vi "PXI-2510 Fault Bus Page.vi"(8 "error in (no error)":errorcluster, 11 "Node Ptr":T2 format="%.0x") -> (0 "error out":errorcluster)   [LabVIEW 2020, in "PXI-2510 System Explorer.lvlib"]
uses:
  PXI-2510 System Explorer.lvlib
  <vilib>/NI VeriStand/Custom Device API/Custom Device Item Ref.ctl
  Shared/Fault Bus Input Selector.ctl
  <vilib>/NI VeriStand/Custom Device API/Custom Device API.lvlib
panel:
  in  "Fault Bus Input Selector Default Value":T1=enum."Input 0"
  in  "Header":cluster{"Section Name":string}={"Section Name"="Custom Device Item Settings"}
  in  "Description":string
  in  "Name":string
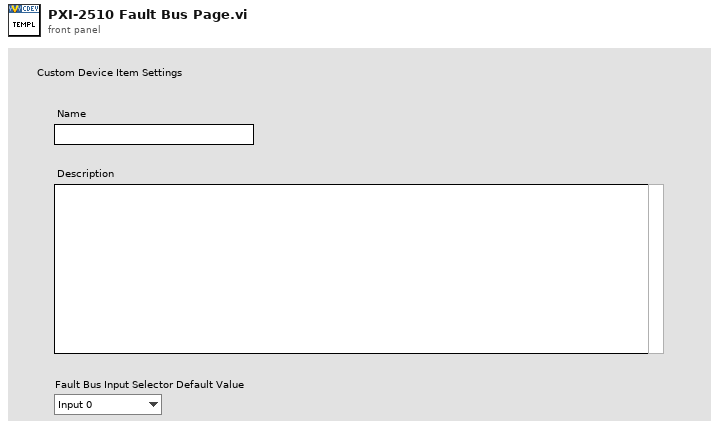
[diagram p1: front panel]
types:
  T1 = typedef "Fault Bus Input Selector.ctl" = enum16{"Default", "Input 0", "Input 1", "Input 2", "Input 3", "Main Bus Only"}
  T2 = typedef "Custom Device API.lvlib/Custom Device Item Ref.ctl" = u64
  T3 = typedef "Custom Device API.lvlib/Custom Device Item Info.ctl" = cluster{"Name":string, "Is Channel":bool, "GUID":string, "Is Waveform":bool}
  T4 = typedef "Custom Device API.lvlib/Custom Device Channel.ctl" = cluster{"Type":T5, "Units":string, "Default Value":dbl, "Faultable":bool, "Scalable":bool}
  T5 = typedef "Custom Device API.lvlib/Custom Device Channel Type.ctl" = enum16{"Input", "Output"}
  T6 = typedef "Custom Device API.lvlib/Custom Device Commands.ctl" = enum16{"Default", "Item renamed", "Shutdown", "Dynamic button pressed"}
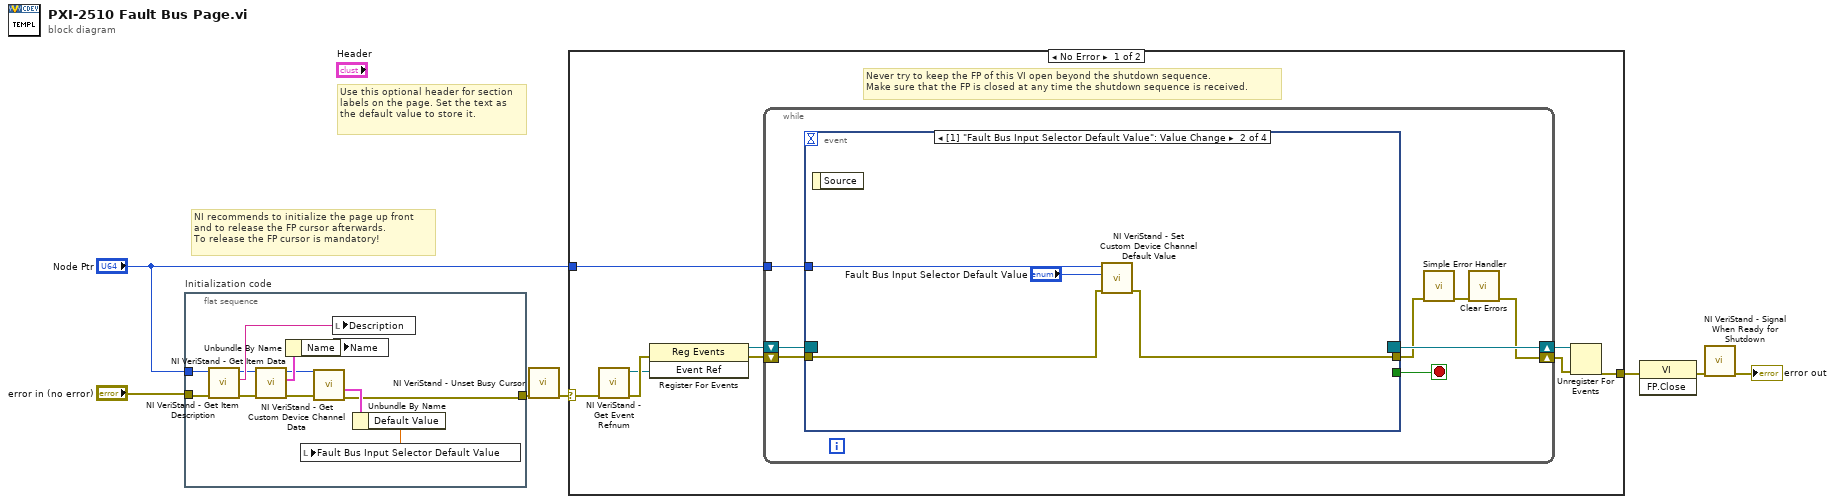
[diagram p0: block diagram]
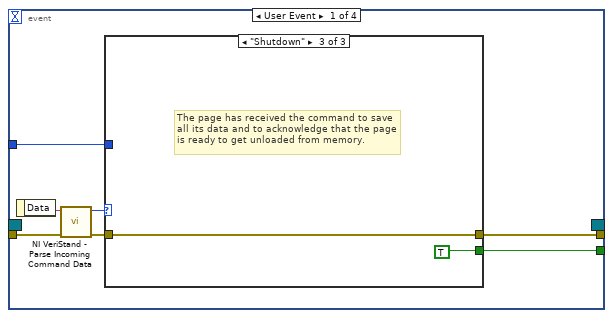
[diagram p2: hidden frame]
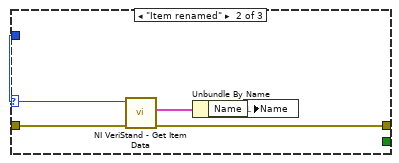
[diagram p4: hidden frame]
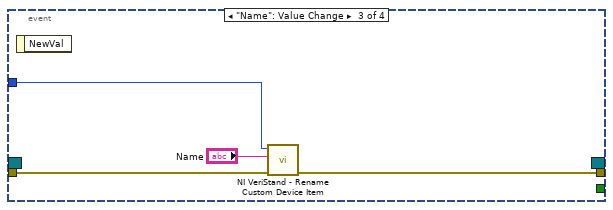
[diagram p5: hidden frame]
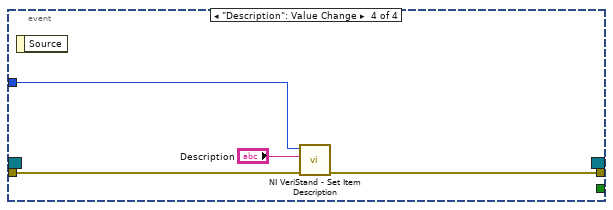
[diagram p6: hidden frame]
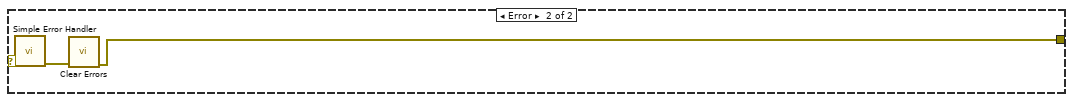
[diagram p7: hidden frame]
diagram:
  # "Use this optional header for section labels on the page. Set the text as the default value to store it."
  # "NI recommends to initialize the page up front\nand to release the FP cursor afterwards.\nTo release the FP cursor is mandatory!"
  n1 = flat-sequence "Initialization code" {
    tunnel: "error in (no error)" -> [w19]
    tunnel: "Node Ptr" -> [w18]
    tunnel: [w8] -> w2
    frame #0 {
      n2 = call <vilib>:"NI VeriStand - Get Item Description.vi"("error in (no error)"=w19, "Item Ref in"=w18) -> ("error out"=w16:errorcluster, "Description"=w17:string, "Item Ref out"=w15:T2)  [unwired: 7 out]
      n3 = call <vilib>:"NI VeriStand - Get Item Data.vi"("error in (no error)"=w16, "Item Ref in"=w15) -> ("error out"=w11:errorcluster, "Item Info"=w14:T3, "Item Ref out"=w12:T2)  [unwired: 7 out]
      n4 = Unbundle By Name(w14) -> ("Name"=w13:string)
      n5 = call <vilib>:"NI VeriStand - Get Custom Device Channel Data.vi"("error in (no error)"=w11, "Channel Ref in"=w12) -> ("error out"=w8:errorcluster, "Channel"=w10:T4)  [unwired: 4 in, 4 out]
      n6 = local write "Description"(w17) -> ()
      n7 = local write "Name"(w13) -> ()
      n8 = Unbundle By Name(w10) -> ("Default Value"=w9:dbl)
      n9 = local write "Fault Bus Input Selector Default Value"(w9) -> ()
    }
  }
  n10 = call <vilib>:"NI VeriStand - Unset Busy Cursor.vi"("error in (no error)"=w2) -> ("error out"=w1:errorcluster)  [unwired: 10 out]
  n11 = case shown="No Error" w1 {
    selector: w1 -> [w20 w66]
    tunnel: [w25 w64] -> w3
    tunnel: "Node Ptr" -> [w21 _]
    frame No Error {
      # "Never try to keep the FP of this VI open beyond the shutdown sequence.\nMake sure that the FP is closed at any time the shutdown sequence is received."
      n12 = call <vilib>:"NI VeriStand - Get Event Refnum.vi"("error in (no error)"=w20) -> ("error out"=w28:errorcluster, "Event Ref"=w24:refnum<user-event>)  [unwired: 9 out]
      n13 = register-events(error in=w28, w24) -> (reference out=w22:refnum<event-registration>, error out=w23:errorcluster)  [unwired: 1 in]
      n14 = while {
        tunnel: w21 -> [w32]
        shift-right: [w29] -> w26
        shift-left: w23 -> [w35]
        shift-right: [w36] -> w27
        shift-left: w22 -> [w34]
        stop <- w33 stop-if-true
        n15 = event shown="[1] \"Fault Bus Input Selector Default Value\": Value Change" {
          selector: w34 -> [_ _ _ _]
          dyn-events: [_ _ _ _] -> w36
          timeout: _ -> [_ _ _ _]
          tunnel: w35 -> [w43 w53 w59 w62]
          tunnel: [w39 _ _ _] -> w33
          tunnel: [w38 w52 w58 w61] -> w31
          tunnel: w32 -> [w37 w55 w57 w63]
          event User Event {
            n16 = event-data() -> ("Data"=w42:string)  [unwired: 1 out]
            n17 = call <vilib>:"NI VeriStand - Parse Incoming Command Data.vi"("error in (no error)"=w43, "Incoming data"=w42) -> ("error out"=w41:errorcluster, "Action"=w40:T6)  [unwired: 8 out]
            n18 = case shown="\"Shutdown\"" w40 {
              tunnel: w41 -> [w44 w49 w50]
              tunnel: [_ _ TRUE] -> w39
              tunnel: [w44 w46 w50] -> w38
              tunnel: w37 -> [_ w48 _]
              frame "Default", Default {
              }
              frame "Item renamed" {
                n19 = call <vilib>:"NI VeriStand - Get Item Data.vi"("error in (no error)"=w49, "Item Ref in"=w48) -> ("error out"=w46:errorcluster, "Item Info"=w47:T3)  [unwired: 8 out]
                n20 = Unbundle By Name(w47) -> ("Name"=w45:string)
                n21 = local write "Name"(w45) -> ()
              }
              frame "Shutdown" {
                # "The page has received the command to save all its data and to acknowledge that the page is ready to get unloaded from memory."
              }
            }
          }
          event Value Change {
            n22 = event-data() -> ()  [unwired: 2 out]
            n23 = call <vilib>:"NI VeriStand - Set Custom Device Channel Default Value.vi"("error in (no error)"=w53, "Default Value"="Fault Bus Input Selector Default Value", "Channel Ref in"=w55) -> ("error out"=w52:errorcluster)  [unwired: 7 in, 1 out]
          }
          event "Name": Value Change {
            n24 = event-data() -> ()  [unwired: 2 out]
            n25 = call <vilib>:"NI VeriStand - Rename Custom Device Item.vi"("error in (no error)"=w59, "New Name"="Name", "Item Ref in"=w57) -> ("error out"=w58:errorcluster)  [unwired: 1 in, 7 out]
          }
          event "Description": Value Change {
            n26 = event-data() -> ()  [unwired: 2 out]
            n27 = call <vilib>:"NI VeriStand - Set Item Description.vi"("error in (no error)"=w62, "Description"="Description", "Item Ref in"=w63) -> ("error out"=w61:errorcluster)  [unwired: 8 out]
          }
        }
        n28 = call <vilib>:"Simple Error Handler.vi"("error in (no error)"=w31) -> ("error out"=w30:errorcluster)  [unwired: 1 in, 7 out]
        n29 = call <vilib>:"Clear Errors.vi"("error in (no error)"=w30) -> ("error out"=w29:errorcluster)  [unwired: 1 in, 5 out]
      }
      n30 = Unregister For Events(event registration refnum=w27, error in=w26) -> (error out=w25:errorcluster)
    }
    frame Error {
      n31 = call <vilib>:"Simple Error Handler.vi"("error in (no error)"=w66) -> ("error out"=w65:errorcluster)  [unwired: 1 in, 7 out]
      n32 = call <vilib>:"Clear Errors.vi"("error in (no error)"=w65) -> ("error out"=w64:errorcluster)  [unwired: 1 in, 5 out]
    }
  }
  n33 = invoke class="VI" method="FP.Close"(error in=w3) -> (error out=w7:errorcluster)  [unwired: 2 in, 2 out]
  n34 = call <vilib>:"NI VeriStand - Signal When Ready for Shutdown.vi"("error in (no error)"=w7) -> ("error out"=→"error out":errorcluster)  [unwired: 10 out]
